vi "Stop Core.vi"(10 "final error code":i32, 11 "CoolAppProcess in":refnum<class "CoolAppProcess.lvclass">) -> (3 "CoolAppProcess out":refnum<class "CoolAppProcess.lvclass">)   [LabVIEW 2020, in "LAF2024Q2.lvlib" / "CoolAppProcess.lvclass"]
doc: "(<B>Filename</B>: Actor Framework.lvlib:Actor.lvclass:Stop Core.vi)\n\nDefines what the actor does before it stops. Use the <B>final error code</B> input to determine whether the actor shut down in response to an error.\n\nBy default, this method passes the Stop message along to all auto-stop nested actors. A descendant class may override this method to define additional behavior, such as shutting down any processes the actor initiated in its override of the Actor Core method."
uses:
  CoolAppProcess.lvclass
  <vilib>/ActorFramework/Actor/Actor.lvclass
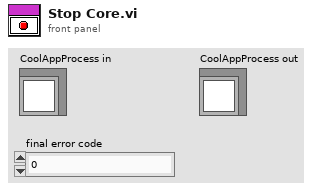
[diagram p1: front panel]
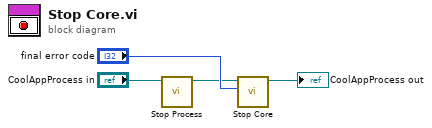
[diagram p0: block diagram]
diagram:
  n1 = call-dynamic "Stop Process.vi"("CoolAppProcess in"="CoolAppProcess in") -> ("CoolAppProcess out"=w1:refnum<class "CoolAppProcess.lvclass">)  [unwired: 9 in, 1 out]
  n2 = call-parent "Stop Core.vi"("final error code"="final error code", "Actor in"=w1) -> ("Actor out"=→"CoolAppProcess out":refnum<class "CoolAppProcess.lvclass">)  [unwired: 9 in]
